vi "NIMS_NS_fir_linfconstr.vi"(5 "Function name":string, 6 "Line number":i32, 7 "Number of outputs requested":i32, 8 "error in (no error)":errorcluster, 11 "[A]":variant[](array[variant])) -> (0 "error out":errorcluster, 3 "[funct(A)]":variant[](array[variant]))   [LabVIEW 2017]
uses:
  <vilib>/imath/engines/lvmath/Functions/Error Handling/error.ctl
  <instcachedir>/0/NIMS_RunTimeType_From StrictType (excl LVString)_1019F277F0A747EDBCA0F6C52CA54500.lvgen/NIMS_RunTimeType_From StrictType (excl LVString)_1019F277F0A747EDBCA0F6C52CA54500_000.vi
  <instcachedir>/0/NIMS_Get Scalar_w Error_1987D997E87247DDAC16EA23A5E9E4FC.lvgen/NIMS_Get Scalar_w Error_1987D997E87247DDAC16EA23A5E9E4FC_000.vi
  <instcachedir>/0/NIMS_Complex To Real_BE01396FDE034E8E94CEBBA1E368668D.lvgen/NIMS_Complex To Real_BE01396FDE034E8E94CEBBA1E368668D_000.vi
  <instcachedir>/0/NIMS_Get Any Vector_w Error - Matrix_9FDB8FBE264C42EDBC8FF9BA66C3EF33.lvgen/NIMS_Get Any Vector_w Error - Matrix_9FDB8FBE264C42EDBC8FF9BA66C3EF33_001.vi
  <instcachedir>/0/NIMS_Get Row Vector_w Error - Matrix_7ECCFA0649AF47C08F6F0C496599EB01.lvgen/NIMS_Get Row Vector_w Error - Matrix_7ECCFA0649AF47C08F6F0C496599EB01_000.vi
  <instcachedir>/0/NIMS_RunTimeType_To Numeric_1CBDAFC4EFAD4045A1DE52278D16738D.lvgen/NIMS_RunTimeType_To Numeric_1CBDAFC4EFAD4045A1DE52278D16738D_000.vi
  <instcachedir>/0/NIMS_Get Row Vector_w Error - Matrix_7ECCFA0649AF47C08F6F0C496599EB01.lvgen/NIMS_Get Row Vector_w Error - Matrix_7ECCFA0649AF47C08F6F0C496599EB01_001.vi
  <vilib>/addons/Digital Filter Design/NI_DigFilter_MathScript.lvlib
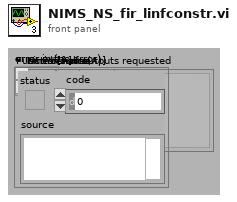
[diagram p1: front panel]
types:
  T1 = typedef "error.ctl" = enum16{"No Error", "Problem", "Input type must not be void", "Incorrect number of parameters", "Function not defined for non-numeric types", "An output variable of the user-defined function is undefined", "Function only defined for character arrays", "Function not defined for boolean, character, or single precision", "Function not defined for complex types", "Not a valid operation", "Inputs must be scalar", "Input matrices are not the same size", "Function only available on RT", "Input matrices must be nonnegative integers of the same type", "Arguments must be non-negative integers less than bitmax", "Number to complement must be less than 2^N", "Bit to get is outside range", "Bit to set is outside range", "Input must be real type ", "At least one parameter must be scalar", "Unable to display plug-in data on RT", "Function not defined for higher dimensional matrices", "Invalid attributes", "Wrong Type of Input Arguments", "Wrong Argument Option", "Invalid file identifier", "Indices must be real positive integers", "The variable is not a matrix data type.", "Number of elements must be the same for indices and values", "You cannot replace elements of a matrix with non-matrix data types.", "Cannot resize a 2D matrix with a linear index", "Unknown variable or symbol", "Indices out of range", "Empty matrix deletion can not be used with two indices", "Number of rows and columns must be the same for indices and values.", "Complex cannot be converted to Boolean", "Char cannot be converted to Boolean", "int64 cannot be converted to Boolean", "uint64 cannot be converted to Boolean", "You cannot convert a Boolean to a character.", "Incompatible input size in 3D surface function", "All rows must have the same number of columns", "Incompatible types", "Invalid matrix dimensions", "Dimension must be 1 or 2", "Base must be an integer between 2 and 36", "Invalid input", "Square matrix required", "Function 'timerstart' must be called before 'timerstop'", "Arguments must be positive real", "Step must not be zero", "Wrong number of input arguments", "Wrong number of output arguments", "Too many index arguments", "Input scalar must be >= 0", "Input scalar must be positive", "Input scalar must not be 0", "Input scalar must be in range [0,1]", "Can't use conditionally defined variable that's undefined", "Input must be a vector", "RT Exec Trace Toolkit not licensed", "Empty vector error", "All elements must be in domain [-1,1]", "All real elements of input vector must be >= 0", "All elements of input vector must be positive", "Values of input vectors are not compatible", "DAQmx not installed", "Input vector must be an increasing vector", "Dereferenced field does not exist within the struct", "A vector or matrix of structures must be indexed before it can be dereferenced", "Lenths of two input vectors are not compatible", "Invalid fieldname", "Empty matrix error", "Cannot use '.' on a type other than Struct", "Unused074", "Data type of the struct's field name is invalid", "Using . to dereference data that is not a struct", "Input struct contains invalid type ", "Size of input matrix is incompatible with input size", "Invalid format specifier", "Could not find field within struct", "Bad permutation array", "Mismatched fieldnames", "ode: User Function could not be opened", "ode: User Function signature does not meet ode requirements", "Unused085", "RunTime: MathScript could not be compiled", "Unknown function", "Only scalars and strings supported", "ode: User Function signature has incorrect number of inputs", "ode:User Function signature has incorrect number of outputs", "Range is too large", "End used without variable", "Function not available (RTE)", "Custom user error", "Arguments must be integers less than bitmax", "Shared library not found", "Header file not found", "Shared library already loaded", "Shared library not loaded", "Shared library function not found", "Shared library string return problem", "Problem calling shared library function", "Problem loading shared library from OS", "Problem parsing shared library header file", "Shared library incompatible types", "Shared library unsupported return type", "Shared library function not exported", "Shared library unsupported input type", "Problem unloading shared library from OS", "Function only available from UI", "Function specified in argument is missing", "An internal error has occurred", "Invalid object", "Invalid property", "Read-only property", "A break command has occurred", "A continue command has occurred", "A return command has occurred", "ode: times parameter invalid", "Function specified in argument has incorrect signature", "Function not found in file", "Reserved keyword cannot be defined as variable", "Reserved keyword cannot be defined as a function or script", "Arguments must be string literals", "Function not supported on this platform", "All columns must have the same number of rows", "Function ignored in RTE warning", "Cannot use : as a parameter that is not a variable", "Output can't be coerced to requested type", "Function not supported on current target", "Variable dependent on an unwired function input", "Unused132", "Unused133", "Unused134", "Unused135", "Unused136", "Unused137", "Unused138", "Unused139", "Global/Persistent must only take constants as arguments.", "Varargin must be last input in the function definition.", "Varargout must be last output in the function definition.", "Invalid output type. Cannot output a cell array of any type other than string.", "Invalid output type. Type is a dynamic struct.", "Invalid output type. Type is a struct that has a field whose type is not known until run-time", "Invalid output type. Type is a struct that has a field which is a plot object.", "MathScript parser DLL missing", "MathScript requires LabVIEW Full", "MathScript license is invalid or missing", "Varargout not supported except in assignments."}
  T2 = typedef "NIMS_CH_character datatype.ctl" = cluster{"Numeric":u8}
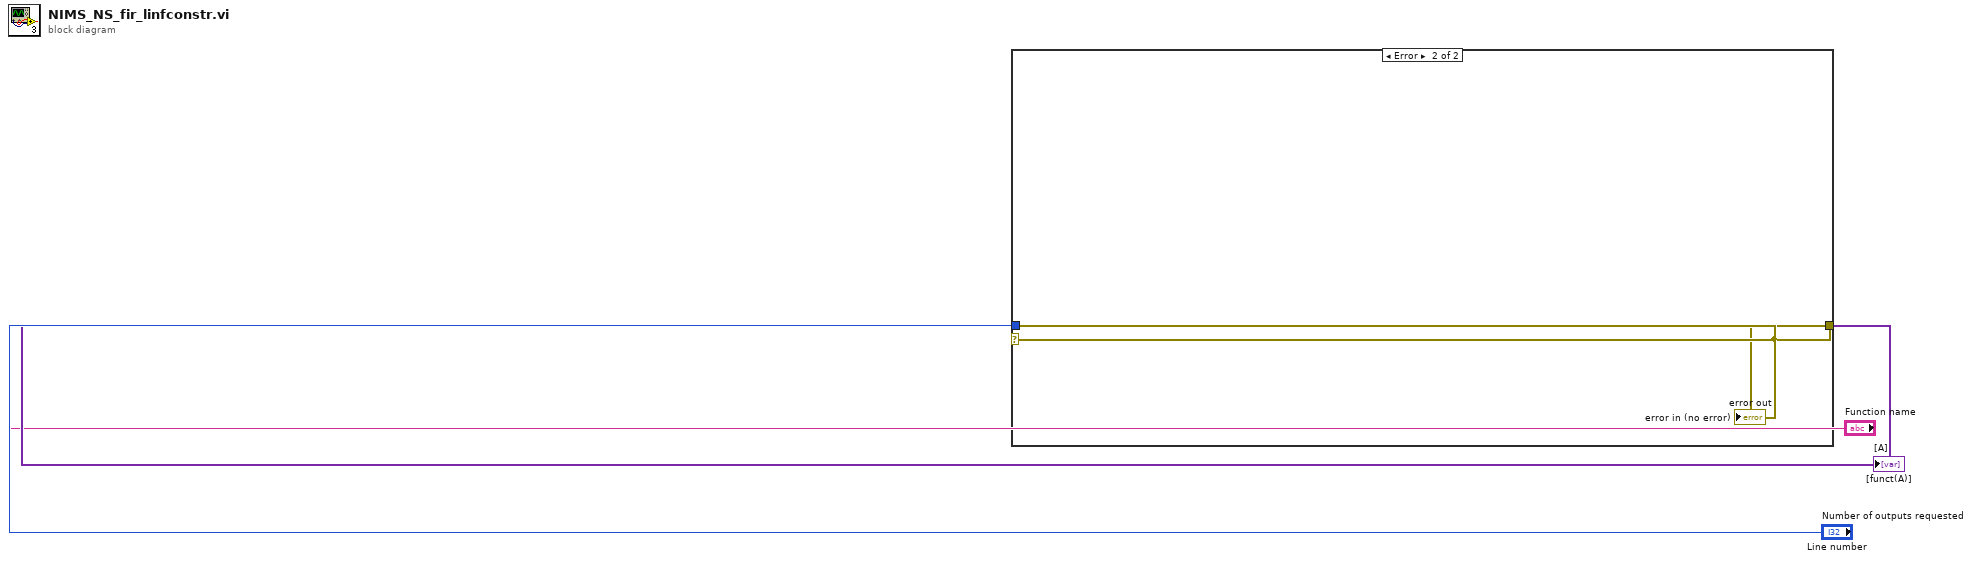
[diagram p0: block diagram]
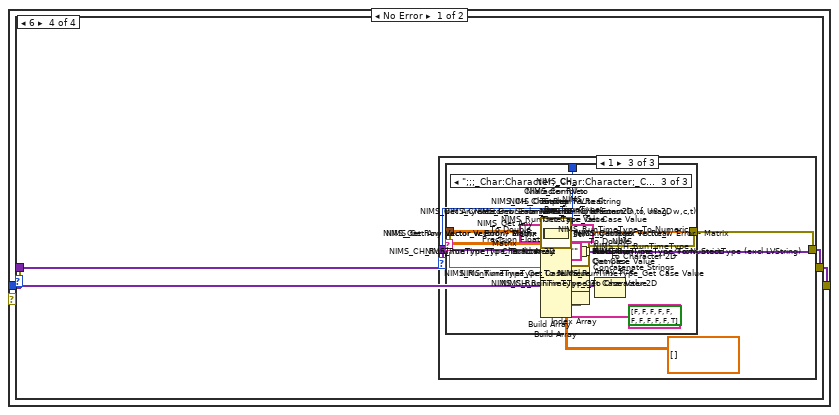
[diagram p2: hidden frame]
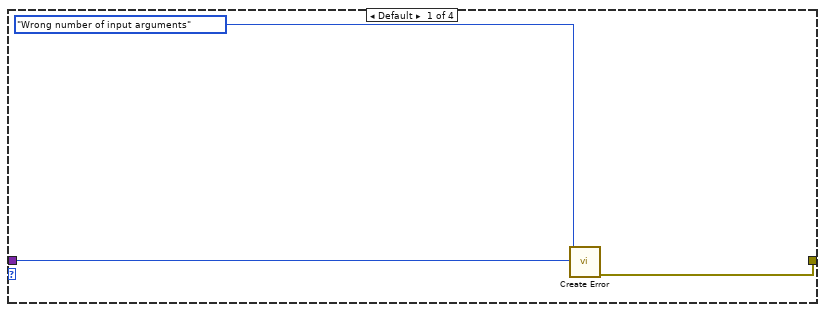
[diagram p3: hidden frame]
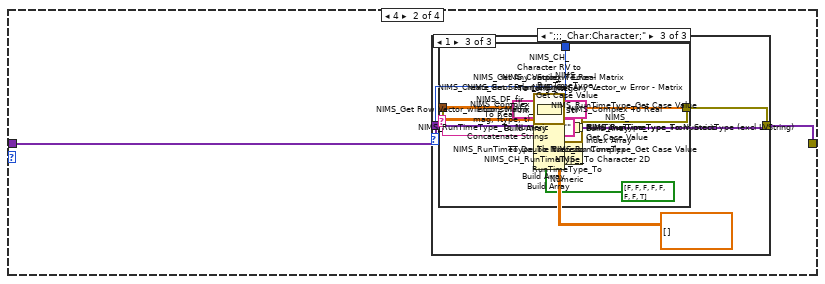
[diagram p4: hidden frame]
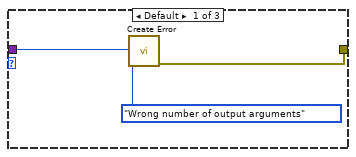
[diagram p5: hidden frame]
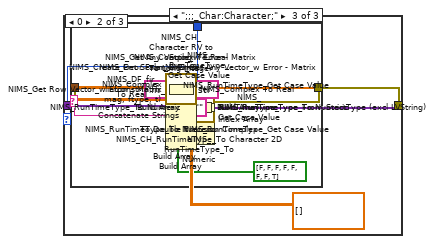
[diagram p6: hidden frame]
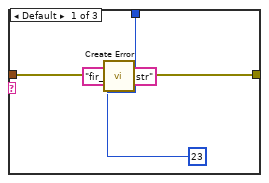
[diagram p7: hidden frame]
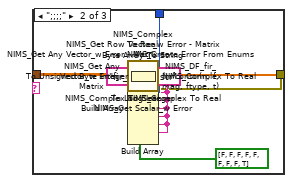
[diagram p8: hidden frame]
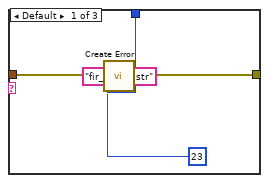
[diagram p9: hidden frame]
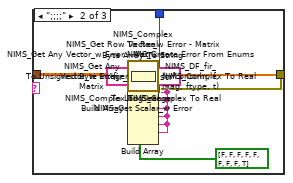
[diagram p10: hidden frame]
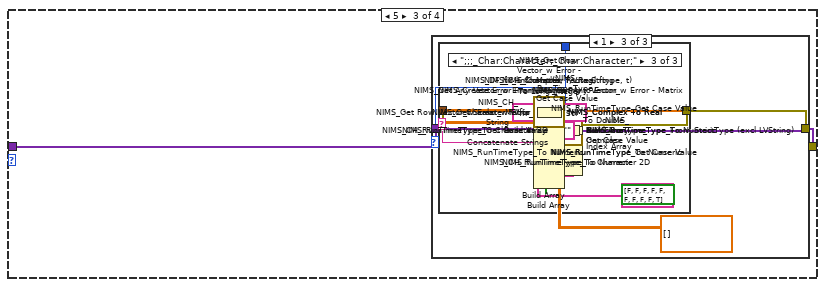
[diagram p11: hidden frame]
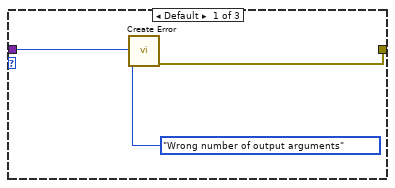
[diagram p12: hidden frame]
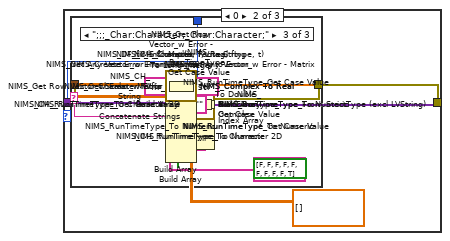
[diagram p13: hidden frame]
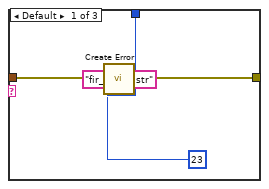
[diagram p14: hidden frame]
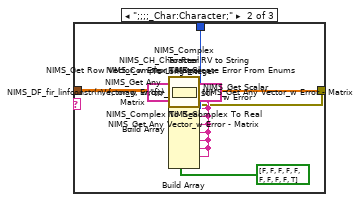
[diagram p15: hidden frame]
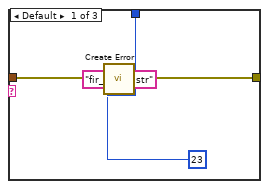
[diagram p16: hidden frame]
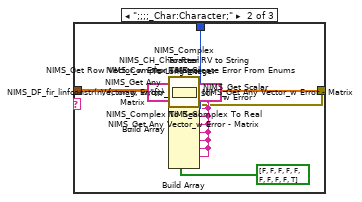
[diagram p17: hidden frame]
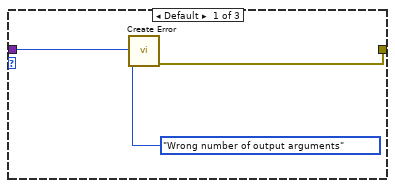
[diagram p18: hidden frame]
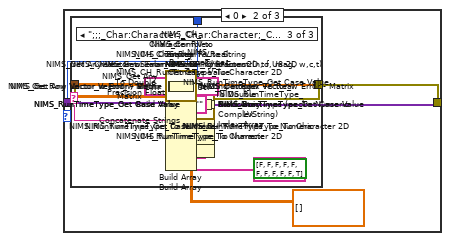
[diagram p19: hidden frame]
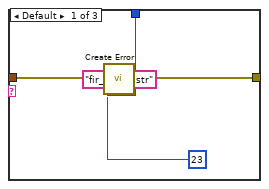
[diagram p20: hidden frame]
diagram:
  n1 = case shown="Error" "error in (no error)" {
    selector: "error in (no error)" -> [_ w711]
    tunnel: [w15 _] -> w4
    tunnel: [w14 w711] -> w3
    tunnel: "error in (no error)" -> [w13 _]
    tunnel: "Number of outputs requested" -> [w12 _]
    tunnel: "[A]" -> [w11 _]
    tunnel: "Function name" -> [w10 _]
    tunnel: "Line number" -> [w9 _]
    frame No Error {
      n2 = Array Size(array=w11) -> (size(s)=w8:i32)
      n3 = case shown="6" w8 {
        tunnel: [_ w27 w231 w459] -> w15
        tunnel: w10 -> [w19 w24 w228 w456]
        tunnel: w9 -> [w20 w25 w229 w457]
        tunnel: w13 -> [w17 w23 w227 w455]
        tunnel: [w16 w22 w226 w454] -> w14
        tunnel: w12 -> [_ w21 w225 w453]
        tunnel: w11 -> [_ w26 w230 w458]
        frame Default {
          n4 = call <vilib>:"Create Error.vi"("Function name"=w19, "error in (no error)"=w17, "Error Enum"=error."Wrong number of input arguments", "Line number"=w20) -> ("error out"=w16:errorcluster)  [unwired: 6 in, 1 out]
        }
        frame 4 {
          n5 = case shown="1" w21 {
            tunnel: [_ w33 w129] -> w27
            tunnel: w24 -> [w31 _ _]
            tunnel: w25 -> [w32 w59 w155]
            tunnel: w23 -> [w29 w57 w153]
            tunnel: [w28 w39 w135] -> w22
            tunnel: w26 -> [_ w60 w156]
            frame Default {
              n6 = call <vilib>:"Create Error.vi"("Function name"=w31, "error in (no error)"=w29, "Error Enum"=error."Wrong number of output arguments", "Line number"=w32) -> ("error out"=w28:errorcluster)  [unwired: 6 in, 1 out]
            }
            frame 0 {
              n7 = Index Array(array=w60) -> (element #1=w56:variant, element #2=w52:variant, element #3=w48:variant, element #4=w44:variant)  [unwired: 4 in]
              n8 = call <vilib>:"NIMS_RunTimeType_Get Case Value.vi"("Data In"=w44) -> ("Case Value"=w40:string)  [unwired: 9 in, 1 out]
              n9 = call <vilib>:"NIMS_CH_RunTimeType_To Character 2D.vi"("Variant"=w44) -> ("data"=w41:T2[][])  [unwired: 1 in]
              n10 = call-generic <vilib>:"NIMS_RunTimeType_To Numeric.vi"("DataType"=cdb[][] [], "Variant"=w44) -> ("data"=w42:cdb[][])  [unwired: 1 in]
              n11 = call <vilib>:"NIMS_RunTimeType_Get Case Value.vi"("Data In"=w48) -> ("Case Value"=w45:string)  [unwired: 9 in, 1 out]
              n12 = call-generic <vilib>:"NIMS_RunTimeType_To Numeric.vi"("DataType"=cdb[][] [], "Variant"=w48) -> ("data"=w46:cdb[][])  [unwired: 1 in]
              n13 = call <vilib>:"NIMS_RunTimeType_Get Case Value.vi"("Data In"=w52) -> ("Case Value"=w49:string)  [unwired: 9 in, 1 out]
              n14 = call-generic <vilib>:"NIMS_RunTimeType_To Numeric.vi"("DataType"=cdb[][] [], "Variant"=w52) -> ("data"=w50:cdb[][])  [unwired: 1 in]
              n15 = call <vilib>:"NIMS_RunTimeType_Get Case Value.vi"("Data In"=w56) -> ("Case Value"=w53:string)  [unwired: 9 in, 1 out]
              n16 = call-generic <vilib>:"NIMS_RunTimeType_To Numeric.vi"("DataType"=cdb[][] [], "Variant"=w56) -> ("data"=w54:cdb[][])  [unwired: 1 in]
              n17 = Concatenate Strings(w53, w49, w45, w40) -> (w58:string)
              n18 = case shown="\";;;_Char:Character;\"" w58 {
                tunnel: w57 -> [w62 w71 w104]
                tunnel: [_ w66 w99] -> w38
                tunnel: [w61 w67 w100] -> w39
                tunnel: w54 -> [_ w97 w127]
                tunnel: w50 -> [_ w93 w123]
                tunnel: w46 -> [_ w90 w120]
                tunnel: w42 -> [_ w87 _]
                tunnel: w41 -> [_ _ w117]
                tunnel: w59 -> [w65 w74 w107]
                frame Default {
                  n19 = call <vilib>:"Create Error.vi"("Function name"="fir_linfconstr", "error in (no error)"=w62, "Error Enum"=23, "Line number"=w65) -> ("error out"=w61:errorcluster)  [unwired: 6 in, 1 out]
                }
                frame ";;;;" {
                  w69 = "fir_linfconstr"
                  n20 = call-generic <vilib>:"NIMS_Complex To Real.vi"("A"=w87) -> ("Error Enum"=w77:T1, "Real(A)"=w86:dbl[][])  [unwired: 8 in, 1 out]
                  n21 = To Unsigned Byte Integer(number=w86) -> (unsigned 8bit integer=w85:u8[][])
                  n22 = call-generic <vilib>:"NIMS_Get Row Vector_w Error - Matrix.vi"("A"=w85) -> ("Error Enum"=w76:T1, "Row Vector"=w84:u8[])  [unwired: 8 in, 1 out]
                  n23 = Byte Array To String(unsigned byte array=w84) -> (string=w88:string)
                  n24 = call-generic <vilib>:"NIMS_Complex To Real.vi"("A"=w90) -> ("Error Enum"=w79:T1, "Real(A)"=w89:dbl[][])  [unwired: 8 in, 1 out]
                  n25 = call-generic <vilib>:"NIMS_Get Any Vector_w Error - Matrix.vi"("A"=w89) -> ("Error Enum"=w78:T1, "Vector"=w91:dbl[])  [unwired: 8 in, 1 out]
                  n26 = call-generic <vilib>:"NIMS_Complex To Real.vi"("A"=w93) -> ("Error Enum"=w81:T1, "Real(A)"=w92:dbl[][])  [unwired: 8 in, 1 out]
                  n27 = call-generic <vilib>:"NIMS_Get Any Vector_w Error - Matrix.vi"("A"=w92) -> ("Error Enum"=w80:T1, "Vector"=w94:dbl[])  [unwired: 8 in, 1 out]
                  n28 = call-generic <vilib>:"NIMS_Complex To Real.vi"("A"=w97) -> ("Error Enum"=w83:T1, "Real(A)"=w96:dbl[][])  [unwired: 8 in, 1 out]
                  n29 = To Long Integer(number=w96) -> (32bit integer=w95:i32[][])
                  n30 = call-generic <vilib>:"NIMS_Get Scalar_w Error.vi"("A"=w95) -> ("Error Enum"=w82:T1, "Scalar"=w98:i32)  [unwired: 8 in, 1 out]
                  n31 = call <vilib>:"NIMS_DF_fir_linfconstr(n, f, mag, ftype, t).vi"("ftype"=w88, "mag"=w91, "f"=w94, "n"=w98) -> ("error"=w75:i32, "b"=w66:dbl[])  [unwired: 6 in]
                  n32 = Build Array(w69, w69, w69, w69, w69, w69, w69, w69, "fir_linfconstr") -> (w72:string[])
                  n33 = Build Array(w83, w82, w81, w80, w79, w78, w77, w76, w75) -> (w73:i32[])
                  n34 = call <vilib>:"NIMS_Create Error From Enums.vi"("Error Code"=bool[] [FALSE, FALSE, FALSE, FALSE, FALSE, FALSE, FALSE, FALSE, TRUE], "error in (no error)"=w71, "Line no"=w74, "Error Enums"=w73, "Function names"=w72) -> ("error out"=w67:errorcluster)  [unwired: 6 in]
                }
                frame ";;;_Char:Character;" {
                  w102 = "fir_linfconstr"
                  n35 = call-generic <vilib>:"NIMS_Get Row Vector_w Error - Matrix.vi"("A"=w117) -> ("Error Enum"=w109:T1, "Row Vector"=w116:T2[])  [unwired: 8 in, 1 out]
                  n36 = call <vilib>:"NIMS_CH_Character RV to String.vi"("Character array"=w116) -> ("String"=w118:string)  [unwired: 10 in]
                  n37 = call-generic <vilib>:"NIMS_Complex To Real.vi"("A"=w120) -> ("Error Enum"=w111:T1, "Real(A)"=w119:dbl[][])  [unwired: 8 in, 1 out]
                  n38 = call-generic <vilib>:"NIMS_Get Any Vector_w Error - Matrix.vi"("A"=w119) -> ("Error Enum"=w110:T1, "Vector"=w121:dbl[])  [unwired: 8 in, 1 out]
                  n39 = call-generic <vilib>:"NIMS_Complex To Real.vi"("A"=w123) -> ("Error Enum"=w113:T1, "Real(A)"=w122:dbl[][])  [unwired: 8 in, 1 out]
                  n40 = call-generic <vilib>:"NIMS_Get Any Vector_w Error - Matrix.vi"("A"=w122) -> ("Error Enum"=w112:T1, "Vector"=w124:dbl[])  [unwired: 8 in, 1 out]
                  n41 = call-generic <vilib>:"NIMS_Complex To Real.vi"("A"=w127) -> ("Error Enum"=w115:T1, "Real(A)"=w126:dbl[][])  [unwired: 8 in, 1 out]
                  n42 = To Long Integer(number=w126) -> (32bit integer=w125:i32[][])
                  n43 = call-generic <vilib>:"NIMS_Get Scalar_w Error.vi"("A"=w125) -> ("Error Enum"=w114:T1, "Scalar"=w128:i32)  [unwired: 8 in, 1 out]
                  n44 = call <vilib>:"NIMS_DF_fir_linfconstr(n, f, mag, ftype, t).vi"("ftype"=w118, "mag"=w121, "f"=w124, "n"=w128) -> ("error"=w108:i32, "b"=w99:dbl[])  [unwired: 6 in]
                  n45 = Build Array(w102, w102, w102, w102, w102, w102, w102, "fir_linfconstr") -> (w105:string[])
                  n46 = Build Array(w115, w114, w113, w112, w111, w110, w109, w108) -> (w106:i32[])
                  n47 = call <vilib>:"NIMS_Create Error From Enums.vi"("Error Code"=bool[] [FALSE, FALSE, FALSE, FALSE, FALSE, FALSE, FALSE, TRUE], "error in (no error)"=w104, "Line no"=w107, "Error Enums"=w106, "Function names"=w105) -> ("error out"=w100:errorcluster)  [unwired: 6 in]
                }
              }
              n48 = Build Array(w38) -> (w37:dbl[][])
              n49 = To Double Precision Complex(1:w37) -> (0:w36:cdb[][])
              n50 = call-generic <vilib>:"NIMS_RunTimeType_From StrictType (excl LVString).vi"("Plug-In Name"="", "Data In"=w36) -> ("Data Out"=w34:variant)  [unwired: 2 in]
              n51 = Build Array(w34) -> (w33:variant[])
            }
            frame 1 {
              n52 = Index Array(array=w156) -> (element #1=w152:variant, element #2=w148:variant, element #3=w144:variant, element #4=w140:variant)  [unwired: 4 in]
              n53 = call <vilib>:"NIMS_RunTimeType_Get Case Value.vi"("Data In"=w140) -> ("Case Value"=w136:string)  [unwired: 9 in, 1 out]
              n54 = call <vilib>:"NIMS_CH_RunTimeType_To Character 2D.vi"("Variant"=w140) -> ("data"=w137:T2[][])  [unwired: 1 in]
              n55 = call-generic <vilib>:"NIMS_RunTimeType_To Numeric.vi"("DataType"=cdb[][] [], "Variant"=w140) -> ("data"=w138:cdb[][])  [unwired: 1 in]
              n56 = call <vilib>:"NIMS_RunTimeType_Get Case Value.vi"("Data In"=w144) -> ("Case Value"=w141:string)  [unwired: 9 in, 1 out]
              n57 = call-generic <vilib>:"NIMS_RunTimeType_To Numeric.vi"("DataType"=cdb[][] [], "Variant"=w144) -> ("data"=w142:cdb[][])  [unwired: 1 in]
              n58 = call <vilib>:"NIMS_RunTimeType_Get Case Value.vi"("Data In"=w148) -> ("Case Value"=w145:string)  [unwired: 9 in, 1 out]
              n59 = call-generic <vilib>:"NIMS_RunTimeType_To Numeric.vi"("DataType"=cdb[][] [], "Variant"=w148) -> ("data"=w146:cdb[][])  [unwired: 1 in]
              n60 = call <vilib>:"NIMS_RunTimeType_Get Case Value.vi"("Data In"=w152) -> ("Case Value"=w149:string)  [unwired: 9 in, 1 out]
              n61 = call-generic <vilib>:"NIMS_RunTimeType_To Numeric.vi"("DataType"=cdb[][] [], "Variant"=w152) -> ("data"=w150:cdb[][])  [unwired: 1 in]
              n62 = Concatenate Strings(w149, w145, w141, w136) -> (w154:string)
              n63 = case shown="\";;;_Char:Character;\"" w154 {
                tunnel: w153 -> [w158 w167 w200]
                tunnel: [_ w162 w195] -> w134
                tunnel: [w157 w163 w196] -> w135
                tunnel: w150 -> [_ w193 w223]
                tunnel: w146 -> [_ w189 w219]
                tunnel: w142 -> [_ w186 w216]
                tunnel: w138 -> [_ w183 _]
                tunnel: w137 -> [_ _ w213]
                tunnel: w155 -> [w161 w170 w203]
                frame Default {
                  n64 = call <vilib>:"Create Error.vi"("Function name"="fir_linfconstr", "error in (no error)"=w158, "Error Enum"=23, "Line number"=w161) -> ("error out"=w157:errorcluster)  [unwired: 6 in, 1 out]
                }
                frame ";;;;" {
                  w165 = "fir_linfconstr"
                  n65 = call-generic <vilib>:"NIMS_Complex To Real.vi"("A"=w183) -> ("Error Enum"=w173:T1, "Real(A)"=w182:dbl[][])  [unwired: 8 in, 1 out]
                  n66 = To Unsigned Byte Integer(number=w182) -> (unsigned 8bit integer=w181:u8[][])
                  n67 = call-generic <vilib>:"NIMS_Get Row Vector_w Error - Matrix.vi"("A"=w181) -> ("Error Enum"=w172:T1, "Row Vector"=w180:u8[])  [unwired: 8 in, 1 out]
                  n68 = Byte Array To String(unsigned byte array=w180) -> (string=w184:string)
                  n69 = call-generic <vilib>:"NIMS_Complex To Real.vi"("A"=w186) -> ("Error Enum"=w175:T1, "Real(A)"=w185:dbl[][])  [unwired: 8 in, 1 out]
                  n70 = call-generic <vilib>:"NIMS_Get Any Vector_w Error - Matrix.vi"("A"=w185) -> ("Error Enum"=w174:T1, "Vector"=w187:dbl[])  [unwired: 8 in, 1 out]
                  n71 = call-generic <vilib>:"NIMS_Complex To Real.vi"("A"=w189) -> ("Error Enum"=w177:T1, "Real(A)"=w188:dbl[][])  [unwired: 8 in, 1 out]
                  n72 = call-generic <vilib>:"NIMS_Get Any Vector_w Error - Matrix.vi"("A"=w188) -> ("Error Enum"=w176:T1, "Vector"=w190:dbl[])  [unwired: 8 in, 1 out]
                  n73 = call-generic <vilib>:"NIMS_Complex To Real.vi"("A"=w193) -> ("Error Enum"=w179:T1, "Real(A)"=w192:dbl[][])  [unwired: 8 in, 1 out]
                  n74 = To Long Integer(number=w192) -> (32bit integer=w191:i32[][])
                  n75 = call-generic <vilib>:"NIMS_Get Scalar_w Error.vi"("A"=w191) -> ("Error Enum"=w178:T1, "Scalar"=w194:i32)  [unwired: 8 in, 1 out]
                  n76 = call <vilib>:"NIMS_DF_fir_linfconstr(n, f, mag, ftype, t).vi"("ftype"=w184, "mag"=w187, "f"=w190, "n"=w194) -> ("error"=w171:i32, "b"=w162:dbl[])  [unwired: 6 in]
                  n77 = Build Array(w165, w165, w165, w165, w165, w165, w165, w165, "fir_linfconstr") -> (w168:string[])
                  n78 = Build Array(w179, w178, w177, w176, w175, w174, w173, w172, w171) -> (w169:i32[])
                  n79 = call <vilib>:"NIMS_Create Error From Enums.vi"("Error Code"=bool[] [FALSE, FALSE, FALSE, FALSE, FALSE, FALSE, FALSE, FALSE, TRUE], "error in (no error)"=w167, "Line no"=w170, "Error Enums"=w169, "Function names"=w168) -> ("error out"=w163:errorcluster)  [unwired: 6 in]
                }
                frame ";;;_Char:Character;" {
                  w198 = "fir_linfconstr"
                  n80 = call-generic <vilib>:"NIMS_Get Row Vector_w Error - Matrix.vi"("A"=w213) -> ("Error Enum"=w205:T1, "Row Vector"=w212:T2[])  [unwired: 8 in, 1 out]
                  n81 = call <vilib>:"NIMS_CH_Character RV to String.vi"("Character array"=w212) -> ("String"=w214:string)  [unwired: 10 in]
                  n82 = call-generic <vilib>:"NIMS_Complex To Real.vi"("A"=w216) -> ("Error Enum"=w207:T1, "Real(A)"=w215:dbl[][])  [unwired: 8 in, 1 out]
                  n83 = call-generic <vilib>:"NIMS_Get Any Vector_w Error - Matrix.vi"("A"=w215) -> ("Error Enum"=w206:T1, "Vector"=w217:dbl[])  [unwired: 8 in, 1 out]
                  n84 = call-generic <vilib>:"NIMS_Complex To Real.vi"("A"=w219) -> ("Error Enum"=w209:T1, "Real(A)"=w218:dbl[][])  [unwired: 8 in, 1 out]
                  n85 = call-generic <vilib>:"NIMS_Get Any Vector_w Error - Matrix.vi"("A"=w218) -> ("Error Enum"=w208:T1, "Vector"=w220:dbl[])  [unwired: 8 in, 1 out]
                  n86 = call-generic <vilib>:"NIMS_Complex To Real.vi"("A"=w223) -> ("Error Enum"=w211:T1, "Real(A)"=w222:dbl[][])  [unwired: 8 in, 1 out]
                  n87 = To Long Integer(number=w222) -> (32bit integer=w221:i32[][])
                  n88 = call-generic <vilib>:"NIMS_Get Scalar_w Error.vi"("A"=w221) -> ("Error Enum"=w210:T1, "Scalar"=w224:i32)  [unwired: 8 in, 1 out]
                  n89 = call <vilib>:"NIMS_DF_fir_linfconstr(n, f, mag, ftype, t).vi"("ftype"=w214, "mag"=w217, "f"=w220, "n"=w224) -> ("error"=w204:i32, "b"=w195:dbl[])  [unwired: 6 in]
                  n90 = Build Array(w198, w198, w198, w198, w198, w198, w198, "fir_linfconstr") -> (w201:string[])
                  n91 = Build Array(w211, w210, w209, w208, w207, w206, w205, w204) -> (w202:i32[])
                  n92 = call <vilib>:"NIMS_Create Error From Enums.vi"("Error Code"=bool[] [FALSE, FALSE, FALSE, FALSE, FALSE, FALSE, FALSE, TRUE], "error in (no error)"=w200, "Line no"=w203, "Error Enums"=w202, "Function names"=w201) -> ("error out"=w196:errorcluster)  [unwired: 6 in]
                }
              }
              n93 = Build Array(w134) -> (w133:dbl[][])
              n94 = To Double Precision Complex(1:w133) -> (0:w132:cdb[][])
              n95 = call-generic <vilib>:"NIMS_RunTimeType_From StrictType (excl LVString).vi"("Plug-In Name"="", "Data In"=w132) -> ("Data Out"=w130:variant)  [unwired: 2 in]
              n96 = Build Array(w130) -> (w129:variant[])
            }
          }
        }
        frame 5 {
          n97 = case shown="1" w225 {
            tunnel: [_ w237 w345] -> w231
            tunnel: w228 -> [w235 _ _]
            tunnel: w229 -> [w236 w266 w374]
            tunnel: w227 -> [w233 w264 w372]
            tunnel: [w232 w243 w351] -> w226
            tunnel: w230 -> [_ w267 w375]
            frame Default {
              n98 = call <vilib>:"Create Error.vi"("Function name"=w235, "error in (no error)"=w233, "Error Enum"=error."Wrong number of output arguments", "Line number"=w236) -> ("error out"=w232:errorcluster)  [unwired: 6 in, 1 out]
            }
            frame 0 {
              n99 = Index Array(array=w267) -> (element #1=w263:variant, element #2=w259:variant, element #3=w255:variant, element #4=w251:variant, element #5=w246:variant)  [unwired: 5 in]
              n100 = call <vilib>:"NIMS_RunTimeType_Get Case Value.vi"("Data In"=w246) -> ("Case Value"=w244:string)  [unwired: 9 in, 1 out]
              n101 = call <vilib>:"NIMS_CH_RunTimeType_To Character 2D.vi"("Variant"=w246) -> ("data"=w245:T2[][])  [unwired: 1 in]
              n102 = call <vilib>:"NIMS_RunTimeType_Get Case Value.vi"("Data In"=w251) -> ("Case Value"=w247:string)  [unwired: 9 in, 1 out]
              n103 = call <vilib>:"NIMS_CH_RunTimeType_To Character 2D.vi"("Variant"=w251) -> ("data"=w248:T2[][])  [unwired: 1 in]
              n104 = call-generic <vilib>:"NIMS_RunTimeType_To Numeric.vi"("DataType"=cdb[][] [], "Variant"=w251) -> ("data"=w249:cdb[][])  [unwired: 1 in]
              n105 = call <vilib>:"NIMS_RunTimeType_Get Case Value.vi"("Data In"=w255) -> ("Case Value"=w252:string)  [unwired: 9 in, 1 out]
              n106 = call-generic <vilib>:"NIMS_RunTimeType_To Numeric.vi"("DataType"=cdb[][] [], "Variant"=w255) -> ("data"=w253:cdb[][])  [unwired: 1 in]
              n107 = call <vilib>:"NIMS_RunTimeType_Get Case Value.vi"("Data In"=w259) -> ("Case Value"=w256:string)  [unwired: 9 in, 1 out]
              n108 = call-generic <vilib>:"NIMS_RunTimeType_To Numeric.vi"("DataType"=cdb[][] [], "Variant"=w259) -> ("data"=w257:cdb[][])  [unwired: 1 in]
              n109 = call <vilib>:"NIMS_RunTimeType_Get Case Value.vi"("Data In"=w263) -> ("Case Value"=w260:string)  [unwired: 9 in, 1 out]
              n110 = call-generic <vilib>:"NIMS_RunTimeType_To Numeric.vi"("DataType"=cdb[][] [], "Variant"=w263) -> ("data"=w261:cdb[][])  [unwired: 1 in]
              n111 = Concatenate Strings(w260, w256, w252, w247, w244) -> (w265:string)
              n112 = case shown="\";;;_Char:Character;_Char:Character;\"" w265 {
                tunnel: w264 -> [w269 w278 w313]
                tunnel: [_ w273 w308] -> w242
                tunnel: [w268 w274 w309] -> w243
                tunnel: w261 -> [_ w306 w343]
                tunnel: w257 -> [_ w302 w339]
                tunnel: w253 -> [_ w299 w336]
                tunnel: w249 -> [_ w296 _]
                tunnel: w248 -> [_ _ w333]
                tunnel: w245 -> [_ w293 w329]
                tunnel: w266 -> [w272 w281 w316]
                frame Default {
                  n113 = call <vilib>:"Create Error.vi"("Function name"="fir_linfconstr", "error in (no error)"=w269, "Error Enum"=23, "Line number"=w272) -> ("error out"=w268:errorcluster)  [unwired: 6 in, 1 out]
                }
                frame ";;;;_Char:Character;" {
                  w276 = "fir_linfconstr"
                  n114 = call-generic <vilib>:"NIMS_Get Row Vector_w Error - Matrix.vi"("A"=w293) -> ("Error Enum"=w283:T1, "Row Vector"=w292:T2[])  [unwired: 8 in, 1 out]
                  n115 = call <vilib>:"NIMS_CH_Character RV to String.vi"("Character array"=w292) -> ("String"=w294:string)  [unwired: 10 in]
                  n116 = call-generic <vilib>:"NIMS_Complex To Real.vi"("A"=w296) -> ("Error Enum"=w285:T1, "Real(A)"=w295:dbl[][])  [unwired: 8 in, 1 out]
                  n117 = call-generic <vilib>:"NIMS_Get Any Vector_w Error - Matrix.vi"("A"=w295) -> ("Error Enum"=w284:T1, "Vector"=w297:dbl[])  [unwired: 8 in, 1 out]
                  n118 = call-generic <vilib>:"NIMS_Complex To Real.vi"("A"=w299) -> ("Error Enum"=w287:T1, "Real(A)"=w298:dbl[][])  [unwired: 8 in, 1 out]
                  n119 = call-generic <vilib>:"NIMS_Get Any Vector_w Error - Matrix.vi"("A"=w298) -> ("Error Enum"=w286:T1, "Vector"=w300:dbl[])  [unwired: 8 in, 1 out]
                  n120 = call-generic <vilib>:"NIMS_Complex To Real.vi"("A"=w302) -> ("Error Enum"=w289:T1, "Real(A)"=w301:dbl[][])  [unwired: 8 in, 1 out]
                  n121 = call-generic <vilib>:"NIMS_Get Any Vector_w Error - Matrix.vi"("A"=w301) -> ("Error Enum"=w288:T1, "Vector"=w303:dbl[])  [unwired: 8 in, 1 out]
                  n122 = call-generic <vilib>:"NIMS_Complex To Real.vi"("A"=w306) -> ("Error Enum"=w291:T1, "Real(A)"=w305:dbl[][])  [unwired: 8 in, 1 out]
                  n123 = To Long Integer(number=w305) -> (32bit integer=w304:i32[][])
                  n124 = call-generic <vilib>:"NIMS_Get Scalar_w Error.vi"("A"=w304) -> ("Error Enum"=w290:T1, "Scalar"=w307:i32)  [unwired: 8 in, 1 out]
                  n125 = call <vilib>:"NIMS_DF_fir_linfconstr(n, f, mag, w,c,t).vi"("c"=w294, "w"=w297, "mag"=w300, "f"=w303, "n"=w307) -> ("error"=w282:i32, "b"=w273:dbl[])  [unwired: 5 in]
                  n126 = Build Array(w276, w276, w276, w276, w276, w276, w276, w276, w276, "fir_linfconstr") -> (w279:string[])
                  n127 = Build Array(w291, w290, w289, w288, w287, w286, w285, w284, w283, w282) -> (w280:i32[])
                  n128 = call <vilib>:"NIMS_Create Error From Enums.vi"("Error Code"=bool[] [FALSE, FALSE, FALSE, FALSE, FALSE, FALSE, FALSE, FALSE, FALSE, TRUE], "error in (no error)"=w278, "Line no"=w281, "Error Enums"=w280, "Function names"=w279) -> ("error out"=w274:errorcluster)  [unwired: 6 in]
                }
                frame ";;;_Char:Character;_Char:Character;" {
                  w311 = "fir_linfconstr"
                  n129 = call-generic <vilib>:"NIMS_Get Row Vector_w Error - Matrix.vi"("A"=w329) -> ("Error Enum"=w319:T1, "Row Vector"=w328:T2[])  [unwired: 8 in, 1 out]
                  n130 = call <vilib>:"NIMS_CH_Character RV to String.vi"("Character array"=w328) -> ("String"=w330:string)  [unwired: 10 in]
                  n131 = call <vilib>:"NIMS_String to Enum.vi"("Input String"=w330, "Enum choices"=string[] ["sym", "antisym", "minphase", "maxphase"] ("Enum Options")) -> ("Error Enum"=w318:T1, "Enum Index"=w331:i32)  [unwired: 8 in]
                  n132 = call-generic <vilib>:"NIMS_Get Row Vector_w Error - Matrix.vi"("A"=w333) -> ("Error Enum"=w320:T1, "Row Vector"=w332:T2[])  [unwired: 8 in, 1 out]
                  n133 = call <vilib>:"NIMS_CH_Character RV to String.vi"("Character array"=w332) -> ("String"=w334:string)  [unwired: 10 in]
                  n134 = call-generic <vilib>:"NIMS_Complex To Real.vi"("A"=w336) -> ("Error Enum"=w322:T1, "Real(A)"=w335:dbl[][])  [unwired: 8 in, 1 out]
                  n135 = call-generic <vilib>:"NIMS_Get Any Vector_w Error - Matrix.vi"("A"=w335) -> ("Error Enum"=w321:T1, "Vector"=w337:dbl[])  [unwired: 8 in, 1 out]
                  n136 = call-generic <vilib>:"NIMS_Complex To Real.vi"("A"=w339) -> ("Error Enum"=w324:T1, "Real(A)"=w338:dbl[][])  [unwired: 8 in, 1 out]
                  n137 = call-generic <vilib>:"NIMS_Get Any Vector_w Error - Matrix.vi"("A"=w338) -> ("Error Enum"=w323:T1, "Vector"=w340:dbl[])  [unwired: 8 in, 1 out]
                  n138 = call-generic <vilib>:"NIMS_Complex To Real.vi"("A"=w343) -> ("Error Enum"=w326:T1, "Real(A)"=w342:dbl[][])  [unwired: 8 in, 1 out]
                  n139 = To Long Integer(number=w342) -> (32bit integer=w341:i32[][])
                  n140 = call-generic <vilib>:"NIMS_Get Scalar_w Error.vi"("A"=w341) -> ("Error Enum"=w325:T1, "Scalar"=w344:i32)  [unwired: 8 in, 1 out]
                  n141 = call <vilib>:"NIMS_DF_fir_linfconstr(n, f, mag, ftype, t).vi"("t"=w331, "ftype"=w334, "mag"=w337, "f"=w340, "n"=w344) -> ("error"=w317:i32, "b"=w308:dbl[])  [unwired: 5 in]
                  n142 = Build Array(w311, w311, w311, w311, w311, w311, w311, w311, w311, "fir_linfconstr") -> (w314:string[])
                  n143 = Build Array(w326, w325, w324, w323, w322, w321, w320, w319, w318, w317) -> (w315:i32[])
                  n144 = call <vilib>:"NIMS_Create Error From Enums.vi"("Error Code"=bool[] [FALSE, FALSE, FALSE, FALSE, FALSE, FALSE, FALSE, FALSE, FALSE, TRUE], "error in (no error)"=w313, "Line no"=w316, "Error Enums"=w315, "Function names"=w314) -> ("error out"=w309:errorcluster)  [unwired: 6 in]
                }
              }
              n145 = Build Array(w242) -> (w241:dbl[][])
              n146 = To Double Precision Complex(1:w241) -> (0:w240:cdb[][])
              n147 = call-generic <vilib>:"NIMS_RunTimeType_From StrictType (excl LVString).vi"("Plug-In Name"="", "Data In"=w240) -> ("Data Out"=w238:variant)  [unwired: 2 in]
              n148 = Build Array(w238) -> (w237:variant[])
            }
            frame 1 {
              n149 = Index Array(array=w375) -> (element #1=w371:variant, element #2=w367:variant, element #3=w363:variant, element #4=w359:variant, element #5=w354:variant)  [unwired: 5 in]
              n150 = call <vilib>:"NIMS_RunTimeType_Get Case Value.vi"("Data In"=w354) -> ("Case Value"=w352:string)  [unwired: 9 in, 1 out]
              n151 = call <vilib>:"NIMS_CH_RunTimeType_To Character 2D.vi"("Variant"=w354) -> ("data"=w353:T2[][])  [unwired: 1 in]
              n152 = call <vilib>:"NIMS_RunTimeType_Get Case Value.vi"("Data In"=w359) -> ("Case Value"=w355:string)  [unwired: 9 in, 1 out]
              n153 = call <vilib>:"NIMS_CH_RunTimeType_To Character 2D.vi"("Variant"=w359) -> ("data"=w356:T2[][])  [unwired: 1 in]
              n154 = call-generic <vilib>:"NIMS_RunTimeType_To Numeric.vi"("DataType"=cdb[][] [], "Variant"=w359) -> ("data"=w357:cdb[][])  [unwired: 1 in]
              n155 = call <vilib>:"NIMS_RunTimeType_Get Case Value.vi"("Data In"=w363) -> ("Case Value"=w360:string)  [unwired: 9 in, 1 out]
              n156 = call-generic <vilib>:"NIMS_RunTimeType_To Numeric.vi"("DataType"=cdb[][] [], "Variant"=w363) -> ("data"=w361:cdb[][])  [unwired: 1 in]
              n157 = call <vilib>:"NIMS_RunTimeType_Get Case Value.vi"("Data In"=w367) -> ("Case Value"=w364:string)  [unwired: 9 in, 1 out]
              n158 = call-generic <vilib>:"NIMS_RunTimeType_To Numeric.vi"("DataType"=cdb[][] [], "Variant"=w367) -> ("data"=w365:cdb[][])  [unwired: 1 in]
              n159 = call <vilib>:"NIMS_RunTimeType_Get Case Value.vi"("Data In"=w371) -> ("Case Value"=w368:string)  [unwired: 9 in, 1 out]
              n160 = call-generic <vilib>:"NIMS_RunTimeType_To Numeric.vi"("DataType"=cdb[][] [], "Variant"=w371) -> ("data"=w369:cdb[][])  [unwired: 1 in]
              n161 = Concatenate Strings(w368, w364, w360, w355, w352) -> (w373:string)
              n162 = case shown="\";;;_Char:Character;_Char:Character;\"" w373 {
                tunnel: w372 -> [w377 w386 w421]
                tunnel: [_ w381 w416] -> w350
                tunnel: [w376 w382 w417] -> w351
                tunnel: w369 -> [_ w414 w451]
                tunnel: w365 -> [_ w410 w447]
                tunnel: w361 -> [_ w407 w444]
                tunnel: w357 -> [_ w404 _]
                tunnel: w356 -> [_ _ w441]
                tunnel: w353 -> [_ w401 w437]
                tunnel: w374 -> [w380 w389 w424]
                frame Default {
                  n163 = call <vilib>:"Create Error.vi"("Function name"="fir_linfconstr", "error in (no error)"=w377, "Error Enum"=23, "Line number"=w380) -> ("error out"=w376:errorcluster)  [unwired: 6 in, 1 out]
                }
                frame ";;;;_Char:Character;" {
                  w384 = "fir_linfconstr"
                  n164 = call-generic <vilib>:"NIMS_Get Row Vector_w Error - Matrix.vi"("A"=w401) -> ("Error Enum"=w391:T1, "Row Vector"=w400:T2[])  [unwired: 8 in, 1 out]
                  n165 = call <vilib>:"NIMS_CH_Character RV to String.vi"("Character array"=w400) -> ("String"=w402:string)  [unwired: 10 in]
                  n166 = call-generic <vilib>:"NIMS_Complex To Real.vi"("A"=w404) -> ("Error Enum"=w393:T1, "Real(A)"=w403:dbl[][])  [unwired: 8 in, 1 out]
                  n167 = call-generic <vilib>:"NIMS_Get Any Vector_w Error - Matrix.vi"("A"=w403) -> ("Error Enum"=w392:T1, "Vector"=w405:dbl[])  [unwired: 8 in, 1 out]
                  n168 = call-generic <vilib>:"NIMS_Complex To Real.vi"("A"=w407) -> ("Error Enum"=w395:T1, "Real(A)"=w406:dbl[][])  [unwired: 8 in, 1 out]
                  n169 = call-generic <vilib>:"NIMS_Get Any Vector_w Error - Matrix.vi"("A"=w406) -> ("Error Enum"=w394:T1, "Vector"=w408:dbl[])  [unwired: 8 in, 1 out]
                  n170 = call-generic <vilib>:"NIMS_Complex To Real.vi"("A"=w410) -> ("Error Enum"=w397:T1, "Real(A)"=w409:dbl[][])  [unwired: 8 in, 1 out]
                  n171 = call-generic <vilib>:"NIMS_Get Any Vector_w Error - Matrix.vi"("A"=w409) -> ("Error Enum"=w396:T1, "Vector"=w411:dbl[])  [unwired: 8 in, 1 out]
                  n172 = call-generic <vilib>:"NIMS_Complex To Real.vi"("A"=w414) -> ("Error Enum"=w399:T1, "Real(A)"=w413:dbl[][])  [unwired: 8 in, 1 out]
                  n173 = To Long Integer(number=w413) -> (32bit integer=w412:i32[][])
                  n174 = call-generic <vilib>:"NIMS_Get Scalar_w Error.vi"("A"=w412) -> ("Error Enum"=w398:T1, "Scalar"=w415:i32)  [unwired: 8 in, 1 out]
                  n175 = call <vilib>:"NIMS_DF_fir_linfconstr(n, f, mag, w,c,t).vi"("c"=w402, "w"=w405, "mag"=w408, "f"=w411, "n"=w415) -> ("error"=w390:i32, "b"=w381:dbl[])  [unwired: 5 in]
                  n176 = Build Array(w384, w384, w384, w384, w384, w384, w384, w384, w384, "fir_linfconstr") -> (w387:string[])
                  n177 = Build Array(w399, w398, w397, w396, w395, w394, w393, w392, w391, w390) -> (w388:i32[])
                  n178 = call <vilib>:"NIMS_Create Error From Enums.vi"("Error Code"=bool[] [FALSE, FALSE, FALSE, FALSE, FALSE, FALSE, FALSE, FALSE, FALSE, TRUE], "error in (no error)"=w386, "Line no"=w389, "Error Enums"=w388, "Function names"=w387) -> ("error out"=w382:errorcluster)  [unwired: 6 in]
                }
                frame ";;;_Char:Character;_Char:Character;" {
                  w419 = "fir_linfconstr"
                  n179 = call-generic <vilib>:"NIMS_Get Row Vector_w Error - Matrix.vi"("A"=w437) -> ("Error Enum"=w427:T1, "Row Vector"=w436:T2[])  [unwired: 8 in, 1 out]
                  n180 = call <vilib>:"NIMS_CH_Character RV to String.vi"("Character array"=w436) -> ("String"=w438:string)  [unwired: 10 in]
                  n181 = call <vilib>:"NIMS_String to Enum.vi"("Input String"=w438, "Enum choices"=string[] ["sym", "antisym", "minphase", "maxphase"] ("Enum Options")) -> ("Error Enum"=w426:T1, "Enum Index"=w439:i32)  [unwired: 8 in]
                  n182 = call-generic <vilib>:"NIMS_Get Row Vector_w Error - Matrix.vi"("A"=w441) -> ("Error Enum"=w428:T1, "Row Vector"=w440:T2[])  [unwired: 8 in, 1 out]
                  n183 = call <vilib>:"NIMS_CH_Character RV to String.vi"("Character array"=w440) -> ("String"=w442:string)  [unwired: 10 in]
                  n184 = call-generic <vilib>:"NIMS_Complex To Real.vi"("A"=w444) -> ("Error Enum"=w430:T1, "Real(A)"=w443:dbl[][])  [unwired: 8 in, 1 out]
                  n185 = call-generic <vilib>:"NIMS_Get Any Vector_w Error - Matrix.vi"("A"=w443) -> ("Error Enum"=w429:T1, "Vector"=w445:dbl[])  [unwired: 8 in, 1 out]
                  n186 = call-generic <vilib>:"NIMS_Complex To Real.vi"("A"=w447) -> ("Error Enum"=w432:T1, "Real(A)"=w446:dbl[][])  [unwired: 8 in, 1 out]
                  n187 = call-generic <vilib>:"NIMS_Get Any Vector_w Error - Matrix.vi"("A"=w446) -> ("Error Enum"=w431:T1, "Vector"=w448:dbl[])  [unwired: 8 in, 1 out]
                  n188 = call-generic <vilib>:"NIMS_Complex To Real.vi"("A"=w451) -> ("Error Enum"=w434:T1, "Real(A)"=w450:dbl[][])  [unwired: 8 in, 1 out]
                  n189 = To Long Integer(number=w450) -> (32bit integer=w449:i32[][])
                  n190 = call-generic <vilib>:"NIMS_Get Scalar_w Error.vi"("A"=w449) -> ("Error Enum"=w433:T1, "Scalar"=w452:i32)  [unwired: 8 in, 1 out]
                  n191 = call <vilib>:"NIMS_DF_fir_linfconstr(n, f, mag, ftype, t).vi"("t"=w439, "ftype"=w442, "mag"=w445, "f"=w448, "n"=w452) -> ("error"=w425:i32, "b"=w416:dbl[])  [unwired: 5 in]
                  n192 = Build Array(w419, w419, w419, w419, w419, w419, w419, w419, w419, "fir_linfconstr") -> (w422:string[])
                  n193 = Build Array(w434, w433, w432, w431, w430, w429, w428, w427, w426, w425) -> (w423:i32[])
                  n194 = call <vilib>:"NIMS_Create Error From Enums.vi"("Error Code"=bool[] [FALSE, FALSE, FALSE, FALSE, FALSE, FALSE, FALSE, FALSE, FALSE, TRUE], "error in (no error)"=w421, "Line no"=w424, "Error Enums"=w423, "Function names"=w422) -> ("error out"=w417:errorcluster)  [unwired: 6 in]
                }
              }
              n195 = Build Array(w350) -> (w349:dbl[][])
              n196 = To Double Precision Complex(1:w349) -> (0:w348:cdb[][])
              n197 = call-generic <vilib>:"NIMS_RunTimeType_From StrictType (excl LVString).vi"("Plug-In Name"="", "Data In"=w348) -> ("Data Out"=w346:variant)  [unwired: 2 in]
              n198 = Build Array(w346) -> (w345:variant[])
            }
          }
        }
        frame 6 {
          n199 = case shown="1" w453 {
            tunnel: [_ w465 w588] -> w459
            tunnel: w456 -> [w463 _ _]
            tunnel: w457 -> [w464 w497 w620]
            tunnel: w455 -> [w461 w495 w618]
            tunnel: [w460 w471 w594] -> w454
            tunnel: w458 -> [_ w498 w621]
            frame Default {
              n200 = call <vilib>:"Create Error.vi"("Function name"=w463, "error in (no error)"=w461, "Error Enum"=error."Wrong number of output arguments", "Line number"=w464) -> ("error out"=w460:errorcluster)  [unwired: 6 in, 1 out]
            }
            frame 0 {
              n201 = Index Array(array=w498) -> (element #1=w494:variant, element #2=w490:variant, element #3=w486:variant, element #4=w482:variant, element #5=w477:variant, element #6=w474:variant)  [unwired: 6 in]
              n202 = call <vilib>:"NIMS_RunTimeType_Get Case Value.vi"("Data In"=w474) -> ("Case Value"=w472:string)  [unwired: 9 in, 1 out]
              n203 = call <vilib>:"NIMS_CH_RunTimeType_To Character 2D.vi"("Variant"=w474) -> ("data"=w473:T2[][])  [unwired: 1 in]
              n204 = call <vilib>:"NIMS_RunTimeType_Get Case Value.vi"("Data In"=w477) -> ("Case Value"=w475:string)  [unwired: 9 in, 1 out]
              n205 = call <vilib>:"NIMS_CH_RunTimeType_To Character 2D.vi"("Variant"=w477) -> ("data"=w476:T2[][])  [unwired: 1 in]
              n206 = call <vilib>:"NIMS_RunTimeType_Get Case Value.vi"("Data In"=w482) -> ("Case Value"=w478:string)  [unwired: 9 in, 1 out]
              n207 = call <vilib>:"NIMS_CH_RunTimeType_To Character 2D.vi"("Variant"=w482) -> ("data"=w479:T2[][])  [unwired: 1 in]
              n208 = call-generic <vilib>:"NIMS_RunTimeType_To Numeric.vi"("DataType"=cdb[][] [], "Variant"=w482) -> ("data"=w480:cdb[][])  [unwired: 1 in]
              n209 = call <vilib>:"NIMS_RunTimeType_Get Case Value.vi"("Data In"=w486) -> ("Case Value"=w483:string)  [unwired: 9 in, 1 out]
              n210 = call-generic <vilib>:"NIMS_RunTimeType_To Numeric.vi"("DataType"=cdb[][] [], "Variant"=w486) -> ("data"=w484:cdb[][])  [unwired: 1 in]
              n211 = call <vilib>:"NIMS_RunTimeType_Get Case Value.vi"("Data In"=w490) -> ("Case Value"=w487:string)  [unwired: 9 in, 1 out]
              n212 = call-generic <vilib>:"NIMS_RunTimeType_To Numeric.vi"("DataType"=cdb[][] [], "Variant"=w490) -> ("data"=w488:cdb[][])  [unwired: 1 in]
              n213 = call <vilib>:"NIMS_RunTimeType_Get Case Value.vi"("Data In"=w494) -> ("Case Value"=w491:string)  [unwired: 9 in, 1 out]
              n214 = call-generic <vilib>:"NIMS_RunTimeType_To Numeric.vi"("DataType"=cdb[][] [], "Variant"=w494) -> ("data"=w492:cdb[][])  [unwired: 1 in]
              n215 = Concatenate Strings(w491, w487, w483, w478, w475, w472) -> (w496:string)
              n216 = case shown="\";;;_Char:Character;_Char:Character;_Char:Character;\"" w496 {
                tunnel: w495 -> [w500 w509 w551]
                tunnel: [_ w504 w546] -> w470
                tunnel: [w499 w505 w547] -> w471
                tunnel: w492 -> [_ w544 w586]
                tunnel: w488 -> [_ w540 w582]
                tunnel: w484 -> [_ w537 w579]
                tunnel: w480 -> [_ w534 _]
                tunnel: w479 -> [_ _ w576]
                tunnel: w476 -> [_ w531 w572]
                tunnel: w473 -> [_ w527 w568]
                tunnel: w497 -> [w503 w512 w554]
                frame Default {
                  n217 = call <vilib>:"Create Error.vi"("Function name"="fir_linfconstr", "error in (no error)"=w500, "Error Enum"=23, "Line number"=w503) -> ("error out"=w499:errorcluster)  [unwired: 6 in, 1 out]
                }
                frame ";;;;_Char:Character;_Char:Character;" {
                  w507 = "fir_linfconstr"
                  n218 = call-generic <vilib>:"NIMS_Get Row Vector_w Error - Matrix.vi"("A"=w527) -> ("Error Enum"=w515:T1, "Row Vector"=w526:T2[])  [unwired: 8 in, 1 out]
                  n219 = call <vilib>:"NIMS_CH_Character RV to String.vi"("Character array"=w526) -> ("String"=w528:string)  [unwired: 10 in]
                  n220 = call <vilib>:"NIMS_String to Enum.vi"("Input String"=w528, "Enum choices"=string[] ["sym", "antisym", "minphase", "maxphase"] ("Enum Options")) -> ("Error Enum"=w514:T1, "Enum Index"=w529:i32)  [unwired: 8 in]
                  n221 = call-generic <vilib>:"NIMS_Get Row Vector_w Error - Matrix.vi"("A"=w531) -> ("Error Enum"=w516:T1, "Row Vector"=w530:T2[])  [unwired: 8 in, 1 out]
                  n222 = call <vilib>:"NIMS_CH_Character RV to String.vi"("Character array"=w530) -> ("String"=w532:string)  [unwired: 10 in]
                  n223 = call-generic <vilib>:"NIMS_Complex To Real.vi"("A"=w534) -> ("Error Enum"=w518:T1, "Real(A)"=w533:dbl[][])  [unwired: 8 in, 1 out]
                  n224 = call-generic <vilib>:"NIMS_Get Any Vector_w Error - Matrix.vi"("A"=w533) -> ("Error Enum"=w517:T1, "Vector"=w535:dbl[])  [unwired: 8 in, 1 out]
                  n225 = call-generic <vilib>:"NIMS_Complex To Real.vi"("A"=w537) -> ("Error Enum"=w520:T1, "Real(A)"=w536:dbl[][])  [unwired: 8 in, 1 out]
                  n226 = call-generic <vilib>:"NIMS_Get Any Vector_w Error - Matrix.vi"("A"=w536) -> ("Error Enum"=w519:T1, "Vector"=w538:dbl[])  [unwired: 8 in, 1 out]
                  n227 = call-generic <vilib>:"NIMS_Complex To Real.vi"("A"=w540) -> ("Error Enum"=w522:T1, "Real(A)"=w539:dbl[][])  [unwired: 8 in, 1 out]
                  n228 = call-generic <vilib>:"NIMS_Get Any Vector_w Error - Matrix.vi"("A"=w539) -> ("Error Enum"=w521:T1, "Vector"=w541:dbl[])  [unwired: 8 in, 1 out]
                  n229 = call-generic <vilib>:"NIMS_Complex To Real.vi"("A"=w544) -> ("Error Enum"=w524:T1, "Real(A)"=w543:dbl[][])  [unwired: 8 in, 1 out]
                  n230 = To Long Integer(number=w543) -> (32bit integer=w542:i32[][])
                  n231 = call-generic <vilib>:"NIMS_Get Scalar_w Error.vi"("A"=w542) -> ("Error Enum"=w523:T1, "Scalar"=w545:i32)  [unwired: 8 in, 1 out]
                  n232 = call <vilib>:"NIMS_DF_fir_linfconstr(n, f, mag, w,c,t).vi"("t"=w529, "c"=w532, "w"=w535, "mag"=w538, "f"=w541, "n"=w545) -> ("error"=w513:i32, "b"=w504:dbl[])  [unwired: 4 in]
                  n233 = Build Array(w507, w507, w507, w507, w507, w507, w507, w507, w507, w507, w507, "fir_linfconstr") -> (w510:string[])
                  n234 = Build Array(w524, w523, w522, w521, w520, w519, w518, w517, w516, w515, w514, w513) -> (w511:i32[])
                  n235 = call <vilib>:"NIMS_Create Error From Enums.vi"("Error Code"=bool[] [FALSE, FALSE, FALSE, FALSE, FALSE, FALSE, FALSE, FALSE, FALSE, FALSE, FALSE, TRUE], "error in (no error)"=w509, "Line no"=w512, "Error Enums"=w511, "Function names"=w510) -> ("error out"=w505:errorcluster)  [unwired: 6 in]
                }
                frame ";;;_Char:Character;_Char:Character;_Char:Character;" {
                  w549 = "fir_linfconstr"
                  n236 = call-generic <vilib>:"NIMS_Get Row Vector_w Error - Matrix.vi"("A"=w568) -> ("Error Enum"=w557:T1, "Row Vector"=w567:T2[])  [unwired: 8 in, 1 out]
                  n237 = call <vilib>:"NIMS_CH_Character RV to String.vi"("Character array"=w567) -> ("String"=w569:string)  [unwired: 10 in]
                  n238 = call <vilib>:"NIMS_String to Enum.vi"("Input String"=w569, "Enum choices"=string[] ["sym", "antisym", "minphase", "maxphase"] ("Enum Options")) -> ("Error Enum"=w556:T1, "Enum Index"=w570:i32)  [unwired: 8 in]
                  n239 = call-generic <vilib>:"NIMS_Get Row Vector_w Error - Matrix.vi"("A"=w572) -> ("Error Enum"=w558:T1, "Row Vector"=w571:T2[])  [unwired: 8 in, 1 out]
                  n240 = call <vilib>:"NIMS_CH_Character RV to String.vi"("Character array"=w571) -> ("String"=w573:string)  [unwired: 10 in]
                  n241 = call <vilib>:"NIMS_CH_Character 2D to U8 2D.vi"("Character 2D array"=w576) -> ("U8 2D array"=w575:u8[][])  [unwired: 10 in]
                  n242 = To Double Precision Float(number=w575) -> (double precision float=w574:dbl[][])
                  n243 = call-generic <vilib>:"NIMS_Get Any Vector_w Error - Matrix.vi"("A"=w574) -> ("Error Enum"=w559:T1, "Vector"=w577:dbl[])  [unwired: 8 in, 1 out]
                  n244 = call-generic <vilib>:"NIMS_Complex To Real.vi"("A"=w579) -> ("Error Enum"=w561:T1, "Real(A)"=w578:dbl[][])  [unwired: 8 in, 1 out]
                  n245 = call-generic <vilib>:"NIMS_Get Any Vector_w Error - Matrix.vi"("A"=w578) -> ("Error Enum"=w560:T1, "Vector"=w580:dbl[])  [unwired: 8 in, 1 out]
                  n246 = call-generic <vilib>:"NIMS_Complex To Real.vi"("A"=w582) -> ("Error Enum"=w563:T1, "Real(A)"=w581:dbl[][])  [unwired: 8 in, 1 out]
                  n247 = call-generic <vilib>:"NIMS_Get Any Vector_w Error - Matrix.vi"("A"=w581) -> ("Error Enum"=w562:T1, "Vector"=w583:dbl[])  [unwired: 8 in, 1 out]
                  n248 = call-generic <vilib>:"NIMS_Complex To Real.vi"("A"=w586) -> ("Error Enum"=w565:T1, "Real(A)"=w585:dbl[][])  [unwired: 8 in, 1 out]
                  n249 = To Long Integer(number=w585) -> (32bit integer=w584:i32[][])
                  n250 = call-generic <vilib>:"NIMS_Get Scalar_w Error.vi"("A"=w584) -> ("Error Enum"=w564:T1, "Scalar"=w587:i32)  [unwired: 8 in, 1 out]
                  n251 = call <vilib>:"NIMS_DF_fir_linfconstr(n, f, mag, w,c,t).vi"("t"=w570, "c"=w573, "w"=w577, "mag"=w580, "f"=w583, "n"=w587) -> ("error"=w555:i32, "b"=w546:dbl[])  [unwired: 4 in]
                  n252 = Build Array(w549, w549, w549, w549, w549, w549, w549, w549, w549, w549, "fir_linfconstr") -> (w552:string[])
                  n253 = Build Array(w565, w564, w563, w562, w561, w560, w559, w558, w557, w556, w555) -> (w553:i32[])
                  n254 = call <vilib>:"NIMS_Create Error From Enums.vi"("Error Code"=bool[] [FALSE, FALSE, FALSE, FALSE, FALSE, FALSE, FALSE, FALSE, FALSE, FALSE, TRUE], "error in (no error)"=w551, "Line no"=w554, "Error Enums"=w553, "Function names"=w552) -> ("error out"=w547:errorcluster)  [unwired: 6 in]
                }
              }
              n255 = Build Array(w470) -> (w469:dbl[][])
              n256 = To Double Precision Complex(1:w469) -> (0:w468:cdb[][])
              n257 = call-generic <vilib>:"NIMS_RunTimeType_From StrictType (excl LVString).vi"("Plug-In Name"="", "Data In"=w468) -> ("Data Out"=w466:variant)  [unwired: 2 in]
              n258 = Build Array(w466) -> (w465:variant[])
            }
            frame 1 {
              n259 = Index Array(array=w621) -> (element #1=w617:variant, element #2=w613:variant, element #3=w609:variant, element #4=w605:variant, element #5=w600:variant, element #6=w597:variant)  [unwired: 6 in]
              n260 = call <vilib>:"NIMS_RunTimeType_Get Case Value.vi"("Data In"=w597) -> ("Case Value"=w595:string)  [unwired: 9 in, 1 out]
              n261 = call <vilib>:"NIMS_CH_RunTimeType_To Character 2D.vi"("Variant"=w597) -> ("data"=w596:T2[][])  [unwired: 1 in]
              n262 = call <vilib>:"NIMS_RunTimeType_Get Case Value.vi"("Data In"=w600) -> ("Case Value"=w598:string)  [unwired: 9 in, 1 out]
              n263 = call <vilib>:"NIMS_CH_RunTimeType_To Character 2D.vi"("Variant"=w600) -> ("data"=w599:T2[][])  [unwired: 1 in]
              n264 = call <vilib>:"NIMS_RunTimeType_Get Case Value.vi"("Data In"=w605) -> ("Case Value"=w601:string)  [unwired: 9 in, 1 out]
              n265 = call <vilib>:"NIMS_CH_RunTimeType_To Character 2D.vi"("Variant"=w605) -> ("data"=w602:T2[][])  [unwired: 1 in]
              n266 = call-generic <vilib>:"NIMS_RunTimeType_To Numeric.vi"("DataType"=cdb[][] [], "Variant"=w605) -> ("data"=w603:cdb[][])  [unwired: 1 in]
              n267 = call <vilib>:"NIMS_RunTimeType_Get Case Value.vi"("Data In"=w609) -> ("Case Value"=w606:string)  [unwired: 9 in, 1 out]
              n268 = call-generic <vilib>:"NIMS_RunTimeType_To Numeric.vi"("DataType"=cdb[][] [], "Variant"=w609) -> ("data"=w607:cdb[][])  [unwired: 1 in]
              n269 = call <vilib>:"NIMS_RunTimeType_Get Case Value.vi"("Data In"=w613) -> ("Case Value"=w610:string)  [unwired: 9 in, 1 out]
              n270 = call-generic <vilib>:"NIMS_RunTimeType_To Numeric.vi"("DataType"=cdb[][] [], "Variant"=w613) -> ("data"=w611:cdb[][])  [unwired: 1 in]
              n271 = call <vilib>:"NIMS_RunTimeType_Get Case Value.vi"("Data In"=w617) -> ("Case Value"=w614:string)  [unwired: 9 in, 1 out]
              n272 = call-generic <vilib>:"NIMS_RunTimeType_To Numeric.vi"("DataType"=cdb[][] [], "Variant"=w617) -> ("data"=w615:cdb[][])  [unwired: 1 in]
              n273 = Concatenate Strings(w614, w610, w606, w601, w598, w595) -> (w619:string)
              n274 = case shown="\";;;_Char:Character;_Char:Character;_Char:Character;\"" w619 {
                tunnel: w618 -> [w623 w632 w674]
                tunnel: [_ w627 w669] -> w593
                tunnel: [w622 w628 w670] -> w594
                tunnel: w615 -> [_ w667 w709]
                tunnel: w611 -> [_ w663 w705]
                tunnel: w607 -> [_ w660 w702]
                tunnel: w603 -> [_ w657 _]
                tunnel: w602 -> [_ _ w699]
                tunnel: w599 -> [_ w654 w695]
                tunnel: w596 -> [_ w650 w691]
                tunnel: w620 -> [w626 w635 w677]
                frame Default {
                  n275 = call <vilib>:"Create Error.vi"("Function name"="fir_linfconstr", "error in (no error)"=w623, "Error Enum"=23, "Line number"=w626) -> ("error out"=w622:errorcluster)  [unwired: 6 in, 1 out]
                }
                frame ";;;;_Char:Character;_Char:Character;" {
                  w630 = "fir_linfconstr"
                  n276 = call-generic <vilib>:"NIMS_Get Row Vector_w Error - Matrix.vi"("A"=w650) -> ("Error Enum"=w638:T1, "Row Vector"=w649:T2[])  [unwired: 8 in, 1 out]
                  n277 = call <vilib>:"NIMS_CH_Character RV to String.vi"("Character array"=w649) -> ("String"=w651:string)  [unwired: 10 in]
                  n278 = call <vilib>:"NIMS_String to Enum.vi"("Input String"=w651, "Enum choices"=string[] ["sym", "antisym", "minphase", "maxphase"] ("Enum Options")) -> ("Error Enum"=w637:T1, "Enum Index"=w652:i32)  [unwired: 8 in]
                  n279 = call-generic <vilib>:"NIMS_Get Row Vector_w Error - Matrix.vi"("A"=w654) -> ("Error Enum"=w639:T1, "Row Vector"=w653:T2[])  [unwired: 8 in, 1 out]
                  n280 = call <vilib>:"NIMS_CH_Character RV to String.vi"("Character array"=w653) -> ("String"=w655:string)  [unwired: 10 in]
                  n281 = call-generic <vilib>:"NIMS_Complex To Real.vi"("A"=w657) -> ("Error Enum"=w641:T1, "Real(A)"=w656:dbl[][])  [unwired: 8 in, 1 out]
                  n282 = call-generic <vilib>:"NIMS_Get Any Vector_w Error - Matrix.vi"("A"=w656) -> ("Error Enum"=w640:T1, "Vector"=w658:dbl[])  [unwired: 8 in, 1 out]
                  n283 = call-generic <vilib>:"NIMS_Complex To Real.vi"("A"=w660) -> ("Error Enum"=w643:T1, "Real(A)"=w659:dbl[][])  [unwired: 8 in, 1 out]
                  n284 = call-generic <vilib>:"NIMS_Get Any Vector_w Error - Matrix.vi"("A"=w659) -> ("Error Enum"=w642:T1, "Vector"=w661:dbl[])  [unwired: 8 in, 1 out]
                  n285 = call-generic <vilib>:"NIMS_Complex To Real.vi"("A"=w663) -> ("Error Enum"=w645:T1, "Real(A)"=w662:dbl[][])  [unwired: 8 in, 1 out]
                  n286 = call-generic <vilib>:"NIMS_Get Any Vector_w Error - Matrix.vi"("A"=w662) -> ("Error Enum"=w644:T1, "Vector"=w664:dbl[])  [unwired: 8 in, 1 out]
                  n287 = call-generic <vilib>:"NIMS_Complex To Real.vi"("A"=w667) -> ("Error Enum"=w647:T1, "Real(A)"=w666:dbl[][])  [unwired: 8 in, 1 out]
                  n288 = To Long Integer(number=w666) -> (32bit integer=w665:i32[][])
                  n289 = call-generic <vilib>:"NIMS_Get Scalar_w Error.vi"("A"=w665) -> ("Error Enum"=w646:T1, "Scalar"=w668:i32)  [unwired: 8 in, 1 out]
                  n290 = call <vilib>:"NIMS_DF_fir_linfconstr(n, f, mag, w,c,t).vi"("t"=w652, "c"=w655, "w"=w658, "mag"=w661, "f"=w664, "n"=w668) -> ("error"=w636:i32, "b"=w627:dbl[])  [unwired: 4 in]
                  n291 = Build Array(w630, w630, w630, w630, w630, w630, w630, w630, w630, w630, w630, "fir_linfconstr") -> (w633:string[])
                  n292 = Build Array(w647, w646, w645, w644, w643, w642, w641, w640, w639, w638, w637, w636) -> (w634:i32[])
                  n293 = call <vilib>:"NIMS_Create Error From Enums.vi"("Error Code"=bool[] [FALSE, FALSE, FALSE, FALSE, FALSE, FALSE, FALSE, FALSE, FALSE, FALSE, FALSE, TRUE], "error in (no error)"=w632, "Line no"=w635, "Error Enums"=w634, "Function names"=w633) -> ("error out"=w628:errorcluster)  [unwired: 6 in]
                }
                frame ";;;_Char:Character;_Char:Character;_Char:Character;" {
                  w672 = "fir_linfconstr"
                  n294 = call-generic <vilib>:"NIMS_Get Row Vector_w Error - Matrix.vi"("A"=w691) -> ("Error Enum"=w680:T1, "Row Vector"=w690:T2[])  [unwired: 8 in, 1 out]
                  n295 = call <vilib>:"NIMS_CH_Character RV to String.vi"("Character array"=w690) -> ("String"=w692:string)  [unwired: 10 in]
                  n296 = call <vilib>:"NIMS_String to Enum.vi"("Input String"=w692, "Enum choices"=string[] ["sym", "antisym", "minphase", "maxphase"] ("Enum Options")) -> ("Error Enum"=w679:T1, "Enum Index"=w693:i32)  [unwired: 8 in]
                  n297 = call-generic <vilib>:"NIMS_Get Row Vector_w Error - Matrix.vi"("A"=w695) -> ("Error Enum"=w681:T1, "Row Vector"=w694:T2[])  [unwired: 8 in, 1 out]
                  n298 = call <vilib>:"NIMS_CH_Character RV to String.vi"("Character array"=w694) -> ("String"=w696:string)  [unwired: 10 in]
                  n299 = call <vilib>:"NIMS_CH_Character 2D to U8 2D.vi"("Character 2D array"=w699) -> ("U8 2D array"=w698:u8[][])  [unwired: 10 in]
                  n300 = To Double Precision Float(number=w698) -> (double precision float=w697:dbl[][])
                  n301 = call-generic <vilib>:"NIMS_Get Any Vector_w Error - Matrix.vi"("A"=w697) -> ("Error Enum"=w682:T1, "Vector"=w700:dbl[])  [unwired: 8 in, 1 out]
                  n302 = call-generic <vilib>:"NIMS_Complex To Real.vi"("A"=w702) -> ("Error Enum"=w684:T1, "Real(A)"=w701:dbl[][])  [unwired: 8 in, 1 out]
                  n303 = call-generic <vilib>:"NIMS_Get Any Vector_w Error - Matrix.vi"("A"=w701) -> ("Error Enum"=w683:T1, "Vector"=w703:dbl[])  [unwired: 8 in, 1 out]
                  n304 = call-generic <vilib>:"NIMS_Complex To Real.vi"("A"=w705) -> ("Error Enum"=w686:T1, "Real(A)"=w704:dbl[][])  [unwired: 8 in, 1 out]
                  n305 = call-generic <vilib>:"NIMS_Get Any Vector_w Error - Matrix.vi"("A"=w704) -> ("Error Enum"=w685:T1, "Vector"=w706:dbl[])  [unwired: 8 in, 1 out]
                  n306 = call-generic <vilib>:"NIMS_Complex To Real.vi"("A"=w709) -> ("Error Enum"=w688:T1, "Real(A)"=w708:dbl[][])  [unwired: 8 in, 1 out]
                  n307 = To Long Integer(number=w708) -> (32bit integer=w707:i32[][])
                  n308 = call-generic <vilib>:"NIMS_Get Scalar_w Error.vi"("A"=w707) -> ("Error Enum"=w687:T1, "Scalar"=w710:i32)  [unwired: 8 in, 1 out]
                  n309 = call <vilib>:"NIMS_DF_fir_linfconstr(n, f, mag, w,c,t).vi"("t"=w693, "c"=w696, "w"=w700, "mag"=w703, "f"=w706, "n"=w710) -> ("error"=w678:i32, "b"=w669:dbl[])  [unwired: 4 in]
                  n310 = Build Array(w672, w672, w672, w672, w672, w672, w672, w672, w672, w672, "fir_linfconstr") -> (w675:string[])
                  n311 = Build Array(w688, w687, w686, w685, w684, w683, w682, w681, w680, w679, w678) -> (w676:i32[])
                  n312 = call <vilib>:"NIMS_Create Error From Enums.vi"("Error Code"=bool[] [FALSE, FALSE, FALSE, FALSE, FALSE, FALSE, FALSE, FALSE, FALSE, FALSE, TRUE], "error in (no error)"=w674, "Line no"=w677, "Error Enums"=w676, "Function names"=w675) -> ("error out"=w670:errorcluster)  [unwired: 6 in]
                }
              }
              n313 = Build Array(w593) -> (w592:dbl[][])
              n314 = To Double Precision Complex(1:w592) -> (0:w591:cdb[][])
              n315 = call-generic <vilib>:"NIMS_RunTimeType_From StrictType (excl LVString).vi"("Plug-In Name"="", "Data In"=w591) -> ("Data Out"=w589:variant)  [unwired: 2 in]
              n316 = Build Array(w589) -> (w588:variant[])
            }
          }
        }
      }
    }
    frame Error {
    }
  }
  "error out" <- w3
  "[funct(A)]" <- w4
